vi "Create Resources.vi"() -> (2 "DIO":refnum<class "Digital IO.lvclass">, 3 "DIO subsystem":refnum<class "Single Address Space Collection.lvclass">)   [LabVIEW 2017, in "Digital IO.lvlib" / "Digital IO.lvclass"]
uses:
  Digital IO.lvclass
  C:/Program Files (x86)/National Instruments/LabVIEW 2017/instr.lib/_niInstr/Instruction Framework/v1/FPGA/Interfaces/Address Space/Address Space.lvclass
  <instrlib>/_niInstr/Instruction Framework/v1/FPGA/Helper Classes/Single Address Space Collection/Single Address Space Collection.lvclass
  <instrlib>/_niInstr/Instruction Framework/v1/FPGA/Interfaces/Address Space/Address Space.lvclass
  Digital IO.lvclass/Digital IO.ctl
  <vilib>/rvi/DataTransferAndStorage/Container/Common/niFpgaContainerGetUniqueNameForEmu.vi
  <vilib>/rvi/DataTransferAndStorage/Container/Common/niFpgaContainerSetEmuInfo.vi
  <vilib>/rvi/eio/common/nirviEmuReportErrorAndStop.vi
  <vilib>/rvi/LocalResourceManager/LocalResourceManager.xnode
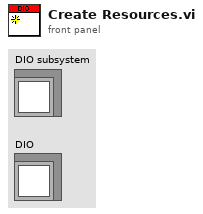
[diagram p1: front panel]
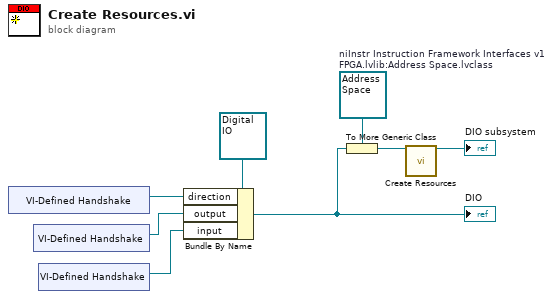
[diagram p0: block diagram]
diagram:
  w6 = refnum<class "Address Space.lvclass"> refnum  # niInstr Instruction Framework Interfaces v1 FPGA.lvlib:Address Space.lvclass
  n1 = xnode "VI-Defined Handshake"() -> ("Handshake Out"=w5:refnum<k21>)
  n2 = xnode "VI-Defined Handshake"() -> ("Handshake Out"=w8:refnum<k21>)
  n3 = xnode "VI-Defined Handshake"() -> ("Handshake Out"=w1:refnum<k21>)
  n4 = Bundle By Name(cluster=refnum<class "Digital IO.lvclass"> refnum ("GPIO"), "direction"=w5, "output"=w8, "input"=w1) -> (w7:refnum<class "Digital IO.lvclass">)
  "DIO" <- w7
  n5 = To More Generic Class(target class=w6, reference=w7) -> (generic class reference=w3:refnum<class "Address Space.lvclass">)
  n6 = call "Create Resources.vi"("address space"=w3) -> ("single address space collection"=→"DIO subsystem":refnum<class "Single Address Space Collection.lvclass">)  [unwired: 14 in]
